vi "Inter_device_ops.vi"(8 "error in (no error)":errorcluster, 9 "UUT Index":i32, 10 "Comm master cluster in":T1={"Main event var"=refnum, "VIRef"=refnum, "Data path"=path "", "Reads"=0, "total number of UUT"=0, "FF refnum"={"Handle1"=0, "Handle2"=0}, "FF device id list"=[], "MODBUS resource name"="", "MODBUS Serial Parameters"={"Mode"=enum."RTU", "Default Slave Address"=0, "MODBUS timeout"=0, "Baud Rate"=0, "Parity"=0, "Flow Control"=0}, "Profibus resource name"="", "Profibus Communication ref.:"=0, "HART resource name"="", "HART long addresses (array)"=[], "Comm relay session"="", "Comm UI event"=refnum, "Write Interval (s)"=5.0, "DMM_QUEUE"=refnum, "POWER_QUEUE"=refnum, "\nTHERM_QUEUE"=refnum, "\nCOMM_QUEUE"=refnum, "TIMING_QUEUE"=refnum, "MAIN_QUEUE"=refnum, "Log path"=path ""} {"Write Interval (s)" min=0.1 max=1000.0 step=0.1}, 11 "Protocol in":refnum<class "Protocol.lvclass">) -> (0 "error out":errorcluster, 3 "Protocol out":refnum<class "Protocol.lvclass">)   [LabVIEW 2016, in "Protocol.lvclass"]
doc: "This is a vi that will do anything required when switching between devices within a cycle. For instance, Profibus requires that a new connection be made to devices with different addresses before a register is interrogated. Etc.."
uses:
  Protocol.lvclass
  MASTER_OPC.ctl
  Typedef/event var.ctl
  Typedef/Comm ui action type.ctl
  Typedef/Comm_State_enum.ctl
  Typedef/state var.ctl
  Protocol.lvclass/Protocol.ctl
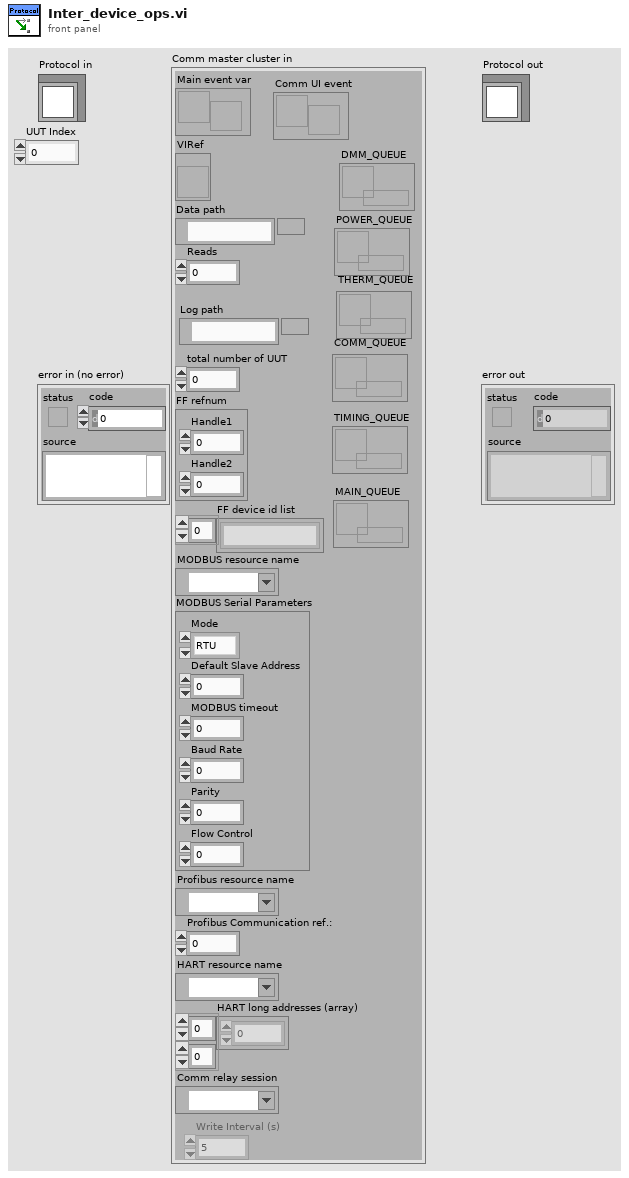
[diagram p1: front panel]
types:
  T1 = typedef "MASTER_OPC.ctl" = cluster{"Main event var":refnum<user-event>, "VIRef":refnum<vi>, "Data path":path, "Reads":i32, "total number of UUT":i32, "FF refnum":cluster{"Handle1":u32, "Handle2":u32}, "FF device id list":string[], "MODBUS resource name":refnum<visa-resource-name>, "MODBUS Serial Parameters":cluster{"Mode":enum16{"RTU", "ASCII"}, "Default Slave Address":u8, "MODBUS timeout":u32, "Baud Rate":u32, "Parity":u16, "Flow Control":u16}, "Profibus resource name":refnum<visa-resource-name>, "Profibus Communication ref.:":u8, "HART resource name":refnum<visa-resource-name>, "HART long addresses (array)":u8[][], "Comm relay session":refnum<k15>, "Comm UI event":refnum<user-event>, "Write Interval (s)":dbl, "DMM_QUEUE":refnum<queue>, "POWER_QUEUE":refnum<queue>, "\nTHERM_QUEUE":refnum<queue>, "\nCOMM_QUEUE":refnum<queue>, "TIMING_QUEUE":refnum<queue>, "MAIN_QUEUE":refnum<queue>, "Log path":path}
  T2 = enum16{"Connect whole bus", "Connect individual UUTs", "Connect none"}
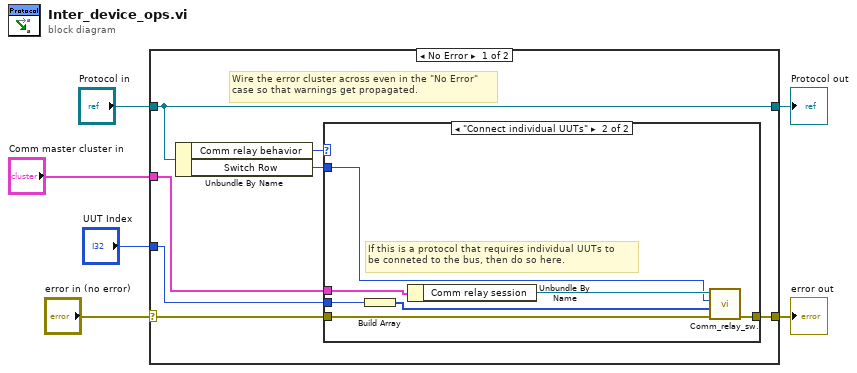
[diagram p0: block diagram]
diagram:
  n1 = case shown="No Error" "error in (no error)" {
    selector: "error in (no error)" -> [w11 w23]
    tunnel: [w10 w23] -> w5
    tunnel: [w13 w22] -> w3
    tunnel: "Protocol in" -> [w13 w22]
    tunnel: "Comm master cluster in" -> [w9 _]
    tunnel: "UUT Index" -> [w8 _]
    frame No Error {
      # "Wire the error cluster across even in the \"No Error\"\ncase so that warnings get propagated."
      n2 = Unbundle By Name(w13) -> ("Comm relay behavior"=w12:T2, "Switch Row"=w7:i32)
      n3 = case shown="\"Connect individual UUTs\"" w12 {
        tunnel: w11 -> [w14 w21]
        tunnel: [w14 w20] -> w10
        tunnel: w9 -> [_ w19]
        tunnel: w8 -> [_ w17]
        tunnel: w7 -> [_ w15]
        frame "Connect whole bus", Default {
        }
        frame "Connect individual UUTs" {
          # "If this is a protocol that requires individual UUTs to \nbe conneted to the bus, then do so here."
          n4 = Build Array(w17) -> (w16:i32[])
          n5 = Unbundle By Name(w19) -> ("Comm relay session"=w18:refnum<k15>)
          n6 = call "Comm_relay_sw..vi"("Error in"=w21, "Columns"=w16, "Row"=w15, "instrument handle in"=w18) -> ("error out"=w20:errorcluster)  [unwired: 6 in, 1 out]
        }
      }
    }
    frame Error {
    }
  }
  "error out" <- w5
  "Protocol out" <- w3
